vi "Measure DAQ Voltages.vi"(8 "error in (no error)":errorcluster, 9 "Averaging":i32=2 min=1, 10 "Descriptions":string[](array[string]), 11 "Array in":refnum<k24>[](array[refnum])) -> (0 "error in (no error) 2":errorcluster, 2 "Raw Voltages":dbl[](array[numeric]), 3 "Array out":refnum<k24>[](array[refnum]), 5 "Sensor Cluster":T1)   [LabVIEW 2016]
uses:
  C:/Cascade-lv16-64/builds/Waterloo Main Program/cascade/data/ULx_LV.dll
  builds/Waterloo Main Program/cascade/data/ULx_LV.dll
  controls/MCC DAQ Readings.ctl
  <vilib>/Analysis/baseanly.llb/Mean (DBL).vi
  <vilib>/ULx/Read.llb/ULx Read (Analog DBL 1Chan 1Samp).vi
  <vilib>/Analysis/NI_AALBase.lvlib
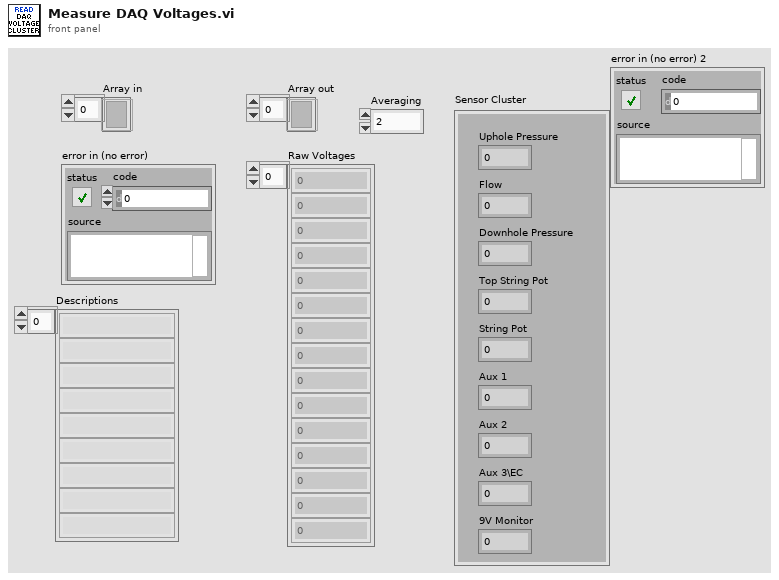
[diagram p1: front panel]
types:
  T1 = typedef "MCC DAQ Readings.ctl" = cluster{"Uphole Pressure":dbl, "Flow":dbl, "Downhole Pressure":dbl, "Top String Pot":dbl, "String Pot":dbl, "Aux 1":dbl, "Aux 2":dbl, "Aux 3\\EC":dbl, "9V Monitor":dbl}
  T2 = cluster{"[0]":dbl, "[1]":dbl, "[2]":dbl, "[3]":dbl, "[4]":dbl, "[5]":dbl, "[6]":dbl, "[7]":dbl, "[8]":dbl}
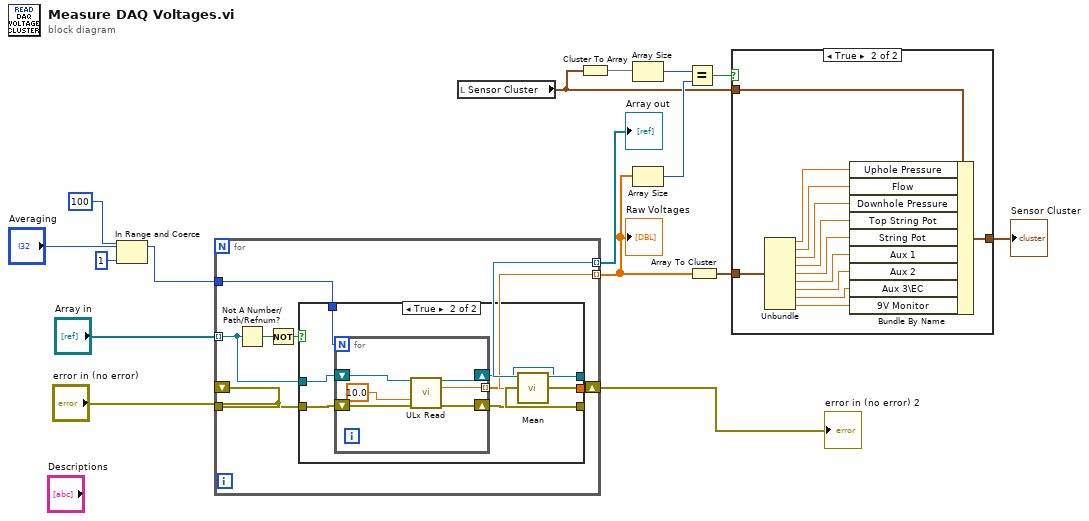
[diagram p0: block diagram]
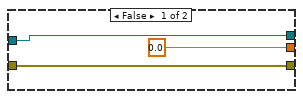
[diagram p3: hidden frame]
diagram:
  n1 = In Range and Coerce(upper limit=100, x="Averaging", lower limit=1) -> (coerced(x)=w3:i32)  [unwired: 1 out]
  n2 = for {
    tunnel: "Array in" -> [w20] mode=indexing
    tunnel: "error in (no error)" -> [w24]
    tunnel: [w23] -> w15 mode=indexing
    tunnel: [w21] -> w9 mode=indexing
    shift-right: [w22] -> w5
    shift-left: "error in (no error)" -> [_]
    tunnel: w3 -> [w17]
    n3 = Not A Number/Path/Refnum?(number/path/refnum=w20) -> (NaN/Path/Refnum?=w19:bool)
    n4 = Not(x=w19) -> (.not. x?=w18:bool)
    n5 = case shown="True" w18 {
      tunnel: w20 -> [w25 w34]
      tunnel: w24 -> [w27 w33]
      tunnel: [w25 w32] -> w23
      tunnel: [w27 w31] -> w22
      tunnel: [0.0 ("data") w28] -> w21
      tunnel: w17 -> [_ w29]
      frame False {
      }
      frame True {
        n6 = for {
          N: w29 -> [_]
          tunnel: [w35] -> w30 mode=indexing
          shift-right: [w37] -> w32
          shift-left: w34 -> [w40]
          shift-right: [w36] -> w31
          shift-left: w33 -> [w39]
          n7 = call-poly <vilib>:"ULx Read.vi"("task in"=w40, "timeout"=10.0, "error in"=w39) -> ("task out"=w37:refnum<k24>, "data"=w35:dbl, "error out"=w36:errorcluster)  [unwired: 10 in]
        }
        n8 = call-poly <vilib>:"Mean.vi"("X"=w30) -> ("mean"=w28:dbl)  [unwired: 1 out]
      }
    }
  }
  "Raw Voltages" <- w9
  "Array out" <- w15
  "error in (no error) 2" <- w5
  n9 = local read "Sensor Cluster"() -> (w6:T1)
  n10 = Cluster To Array(cluster=w6) -> (array=w13:dbl[])
  n11 = Array Size(array=w13) -> (size(s)=w11:i32)
  n12 = Array Size(array=w9) -> (size(s)=w10:i32)
  n13 = Equal?(x=w11, y=w10) -> (x = y?=w12:bool)
  n14 = Array To Cluster(array=w9) -> (cluster=w8:T2)
  n15 = case shown="True" w12 {
    tunnel: [w41 w53] -> w7
    tunnel: w6 -> [w41 w52]
    tunnel: w8 -> [_ w51]
    frame False {
    }
    frame True {
      n16 = Unbundle(w51) -> ("[0]"=w50:dbl, "[1]"=w49:dbl, "[2]"=w48:dbl, "[3]"=w47:dbl, "[4]"=w46:dbl, "[5]"=w45:dbl, "[6]"=w44:dbl, "[7]"=w43:dbl, "[8]"=w42:dbl)
      n17 = Bundle By Name(cluster=w52, "Uphole Pressure"=w50, "Flow"=w49, "Downhole Pressure"=w48, "Top String Pot"=w47, "String Pot"=w46, "Aux 1"=w45, "Aux 2"=w44, "Aux 3\\EC"=w43, "9V Monitor"=w42) -> (w53:T1)
    }
  }
  "Sensor Cluster" <- w7
